vi "Write LLP Packets to CSI-2 TX Buffer.vi"(0 "tagged llp packet":T1, 1 "reset":bool, 2 "resources":T10, 5 "generate packet":bool, 9 "input valid":bool) -> (4 "ready to generate packet":bool, 6 "num packets in tx buffer":fxp<+,14,14>, 8 "num generated packets":u64, 14 "ready for input":bool)   [LabVIEW 2020, in "GettingStarted_Gen_148X_FPGA.lvlib"]
uses:
  GettingStarted_Gen_148X_FPGA.lvlib
  <instrlib>/FlexRIO/CSI-2/v2/FPGA/NI CSI-2 API FPGA v2.lvlib
  Common/Types/Serial Output Channel IO.ctl
  Common/GettingStarted_Common_148X_FPGA.lvlib
  Common/Types/I2C IO.ctl
  Types/Serial Output Channel Resources.ctl
  <instrlib>/FlexRIO/CSI-2/v2/FPGA/Types/LLP Packet Header.ctl
  <instrlib>/FlexRIO/CSI-2/v2/FPGA/Types/LLP Packet Payload.ctl
  <instrlib>/FlexRIO/CSI-2/v2/FPGA/Types/LLP Packet Footer.ctl
  <instrlib>/FlexRIO/CSI-2/v2/FPGA/Types/LLP Packet.ctl
  <instrlib>/FlexRIO/CSI-2/v2/FPGA/Types/Timestamp ID.ctl
  <instrlib>/FlexRIO/CSI-2/v2/FPGA/Types/FPGA LLP Packet Timestamp.ctl
  <instrlib>/FlexRIO/CSI-2/v2/FPGA/Types/FPGA LLP Packet Size.ctl
  <instrlib>/FlexRIO/CSI-2/v2/FPGA/Types/FPGA LLP Packet Tag.ctl
  <instrlib>/FlexRIO/CSI-2/v2/FPGA/Types/Tagged LLP Packet.ctl
  Common/Types/Single Serial Channel Resources.ctl
  Common/Types/Serial Output Channel IO 32b.ctl
  Common/Types/Serial Output Channel IO 64b.ctl
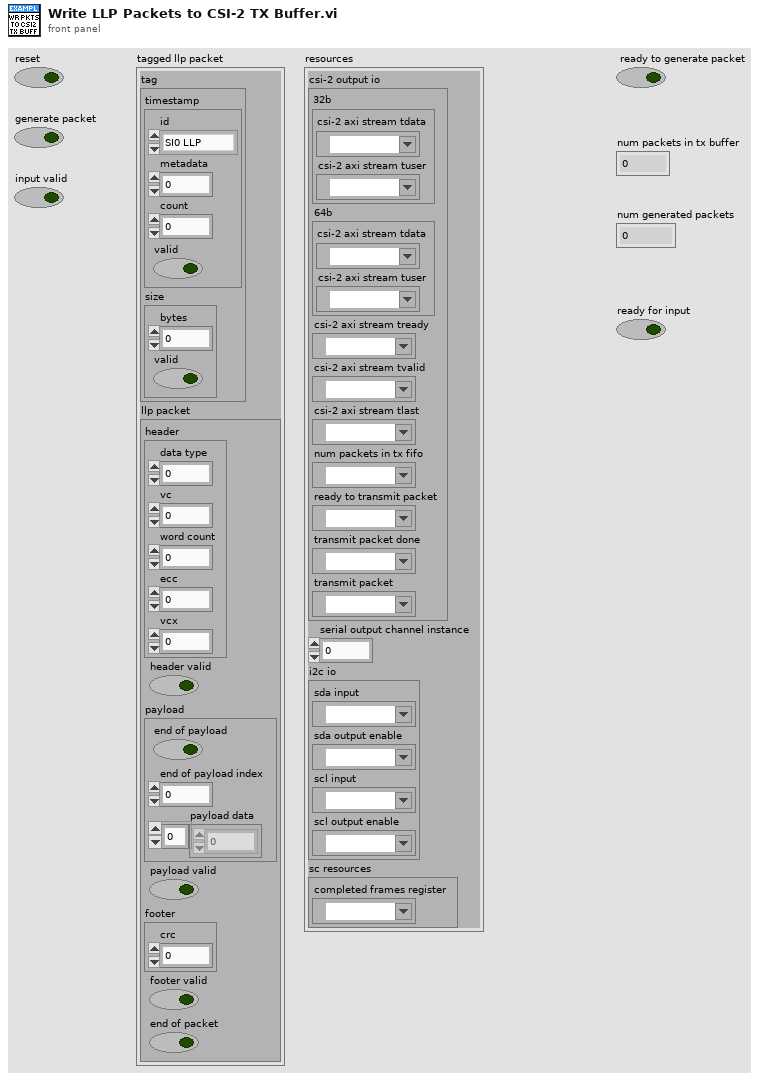
[diagram p1: front panel]
types:
  T1 = typedef "NI CSI-2 API FPGA v2.lvlib/Tagged LLP Packet.ctl" = cluster{"tag":T2, "llp packet":T6}
  T2 = typedef "NI CSI-2 API FPGA v2.lvlib/FPGA LLP Packet Tag.ctl" = cluster{"timestamp":T3, "size":T5}
  T3 = typedef "NI CSI-2 API FPGA v2.lvlib/FPGA LLP Packet Timestamp.ctl" = cluster{"valid":bool, "count":fxp<+,50,50>, "id":T4, "metadata":u8}
  T4 = typedef "NI CSI-2 API FPGA v2.lvlib/Timestamp ID.ctl" = enum8{"SI0 LLP", "SI1 LLP", "SI2 LLP", "SI3 LLP", "SI4 LLP", "SI5 LLP", "SI6 LLP", "SI7 LLP", "SO0 LLP", "SO1 LLP", "SO2 LLP", "SO3 LLP", "SO4 LLP", "SO5 LLP", "SO6 LLP", "SO7 LLP", "Ser0 GPIO Bank", "Ser1 GPIO Bank", "Ser2 GPIO Bank", "Ser3 GPIO Bank", "Ser4 GPIO Bank", "Ser5 GPIO Bank", "Ser6 GPIO Bank", "Ser7 GPIO Bank", "Des0 GPIO Bank", "Des1 GPIO Bank", "Des2 GPIO Bank", "Des3 GPIO Bank", "Des4 GPIO Bank", "Des5 GPIO Bank", "Des6 GPIO Bank", "Des7 GPIO Bank", "User0", "User1", "User2", "User3", "User4", "User5", "User6", "User7", "User8", "User9", "User10", "User11", "User12", "User13", "User14", "User15", "User16", "User17", "User18", "User19", "User20", "User21", "User22", "User23", "User24", "User25", "User26", "User27", "User28", "User29", "User30", "User31"}
  T5 = typedef "NI CSI-2 API FPGA v2.lvlib/FPGA LLP Packet Size.ctl" = cluster{"bytes":fxp<+,17,17>, "valid":bool}
  T6 = typedef "NI CSI-2 API FPGA v2.lvlib/LLP Packet.ctl" = cluster{"header":T7, "header valid":bool, "payload":T8, "payload valid":bool, "footer":T9, "footer valid":bool, "end of packet":bool}
  T7 = typedef "NI CSI-2 API FPGA v2.lvlib/LLP Packet Header.ctl" = cluster{"word count":u16, "ecc":fxp<+,6,6>, "vcx":fxp<+,2,2>, "data type":fxp<+,6,6>, "vc":fxp<+,2,2>}
  T8 = typedef "NI CSI-2 API FPGA v2.lvlib/LLP Packet Payload.ctl" = cluster{"end of payload":bool, "end of payload index":fxp<+,3,3>, "payload data":u8[]}
  T9 = typedef "NI CSI-2 API FPGA v2.lvlib/LLP Packet Footer.ctl" = cluster{"crc":u16}
  T10 = typedef "GettingStarted_Gen_148X_FPGA.lvlib/Serial Output Channel Resources.ctl" = cluster{"csi-2 output io":T11, "serial output channel instance":u8, "i2c io":T14, "sc resources":T15}
  T11 = typedef "GettingStarted_Common_148X_FPGA.lvlib/Serial Output Channel IO.ctl" = cluster{"32b":T12, "64b":T13, "csi-2 axi stream tready":refnum<k21>, "csi-2 axi stream tvalid":refnum<k21>, "csi-2 axi stream tlast":refnum<k21>, "num packets in tx fifo":refnum<k21>, "ready to transmit packet":refnum<k21>, "transmit packet done":refnum<k21>, "transmit packet":refnum<k21>}
  T12 = typedef "GettingStarted_Common_148X_FPGA.lvlib/Serial Output Channel IO 32b.ctl" = cluster{"csi-2 axi stream tdata":refnum<k21>, "csi-2 axi stream tuser":refnum<k21>}
  T13 = typedef "GettingStarted_Common_148X_FPGA.lvlib/Serial Output Channel IO 64b.ctl" = cluster{"csi-2 axi stream tdata":refnum<k21>, "csi-2 axi stream tuser":refnum<k21>}
  T14 = typedef "GettingStarted_Common_148X_FPGA.lvlib/I2C IO.ctl" = cluster{"sda input":refnum<k21>, "sda output enable":refnum<k21>, "scl input":refnum<k21>, "scl output enable":refnum<k21>}
  T15 = typedef "GettingStarted_Common_148X_FPGA.lvlib/Single Serial Channel Resources.ctl" = cluster{"completed frames register":refnum<k21>}
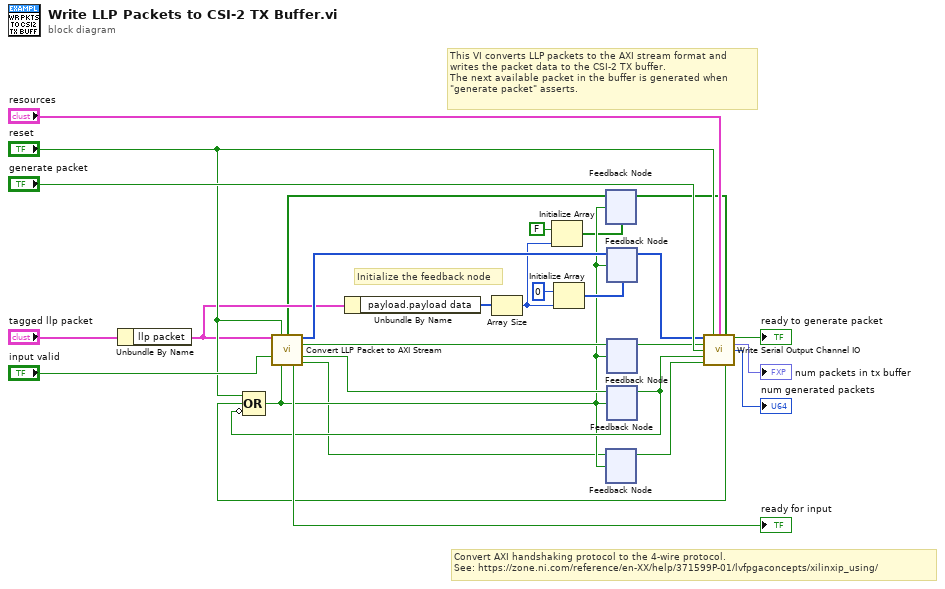
[diagram p0: block diagram]
diagram:
  # "Initialize the feedback node"
  # "Convert AXI handshaking protocol to the 4-wire protocol.\nSee: https://zone.ni.com/reference/en-XX/help/371599P-01/lvfpgaconcepts/xilinxip_using/"
  # "This VI converts LLP packets to the AXI stream format and \nwrites the packet data to the CSI-2 TX buffer. \nThe next available packet in the buffer is generated when \n\"generate packet\" asserts."
  n1 = Unbundle By Name("tagged llp packet") -> ("llp packet"=w9:T6)
  n2 = Unbundle By Name(w9) -> ("payload.payload data"=w11:u8[])
  n3 = Array Size(array=w11) -> (size(s)=w3:i32)
  n4 = Initialize Array(FALSE ("filler valid"), w3) -> (w2:bool[])
  n5 = Initialize Array(u8 0 ("element"), w3) -> (w10:u8[])
  n6 = feedback #1(w2) -> (w5:bool[])
  n7 = feedback #2() -> (w8:bool)  [unwired: 1 in]
  n8 = feedback #3(w10) -> (w16:u8[])
  n9 = feedback #4() -> (w17:bool)  [unwired: 1 in]
  n10 = feedback #5() -> (w19:bool)  [unwired: 1 in]
  n11 = call "Write Serial Output Channel IO.vi"("packet word"=w16, "reset"="reset", "resources"="resources", "filler valid"=w5, "end of packet"=w17, "generate packet"="generate packet", "input valid"=w19, "header valid"=w8) -> ("ready to generate packet"=→"ready to generate packet":bool, "num packets in tx buffer"=→"num packets in tx buffer":fxp<+,14,14>, "num generated packets"=→"num generated packets":u64, "tready"=w15:bool)  [unwired: 4 in]
  n12 = Compound Arithmetic op=OR("reset", w15, invert w19) -> (w7:bool)
  n13 = call <instrlib>:"Convert LLP Packet to AXI Stream.vi"("llp packet"=w9, "reset"="reset", "input valid"="input valid", "ready for output"=w7) -> ("filler valid"=w6:bool[], "packet word"=w13:u8[], "end of packet"=w18:bool, "output valid"=w20:bool, "ready for input"=→"ready for input":bool, "header valid"=w1:bool)  [unwired: 6 in]
  n14 = feedback-in #1(w6, w7) -> ()
  n15 = feedback-in #2(w1, w7) -> ()
  n16 = feedback-in #3(w13, w7) -> ()
  n17 = feedback-in #4(w18, w7) -> ()
  n18 = feedback-in #5(w20, w7) -> ()
